vi "Colum_Auto_Size.vi"(8 "error in (no error)":errorcluster, 10 "Table With header":string[][](array[string])=[["", ""], ["", ""]], 11 "Table reference":refnum<vi>) -> (0 "error out":errorcluster)   [LabVIEW 2017]
doc: "This Vi is Created by Asim Lambay for auto sizing of Table Colum. Please use header also with it."
uses:
  <vilib>/Utility/miscctls.llb/LVRowAndColumnTypeDef.ctl
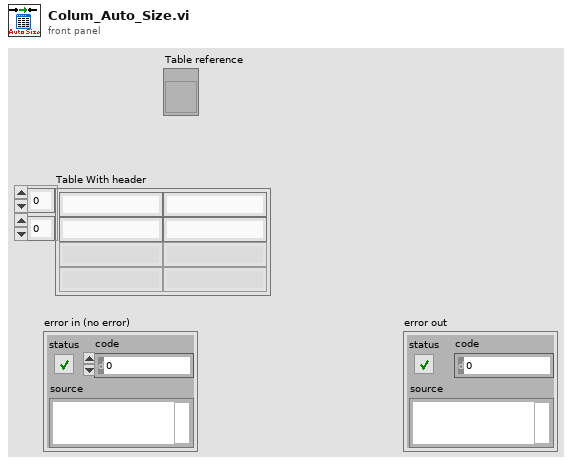
[diagram p1: front panel]
types:
  T1 = typedef "LVRowAndColumnTypeDef.ctl" = cluster{"Row":i32, "Column":i32}
  T2 = typedef "LVBoundsTypeDef.ctl" = cluster{"Width":u32, "Height":u32}
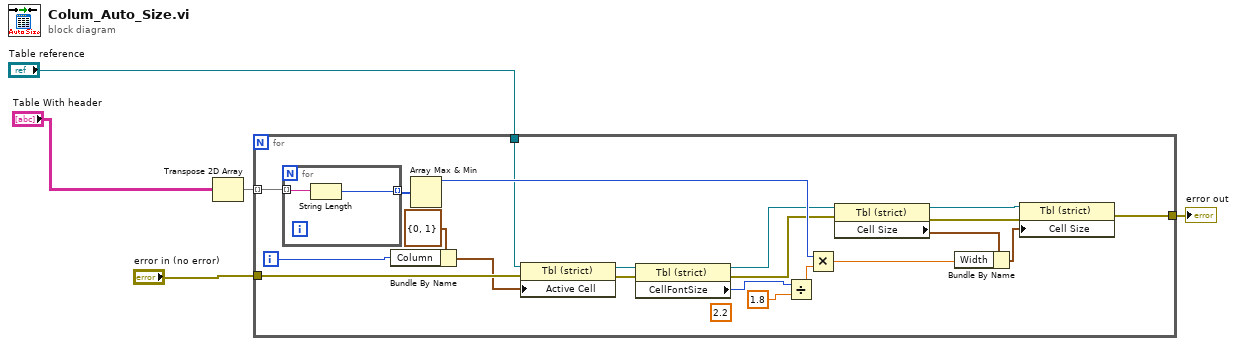
[diagram p0: block diagram]
diagram:
  n1 = Transpose 2D Array(2D array="Table With header") -> (transposed array=w4:string[][])
  n2 = for {
    tunnel: w4 -> [w26] mode=indexing
    tunnel: "error in (no error)" -> [w22]
    tunnel: [w8] -> w2
    tunnel: "Table reference" -> [w7]
    i -> [w23]
    (unwired) 2.2 ("x/y 2")
    n3 = for {
      tunnel: w26 -> [w28] mode=indexing
      tunnel: [w27] -> w25 mode=indexing
      n4 = String Length(string=w28) -> (length=w27:i32)
    }
    n5 = Bundle By Name(cluster=T1 {"Row"=0, "Column"=1} ("Active Cel"), "Column"=w23) -> (w21:T1)
    n6 = Array Max & Min(array=w25) -> (max value=w16:i32)  [unwired: 3 out]
    n7 = property on="Property Node" class="Tbl (strict)"(reference=w7, error in=w22, "Active Cell"=w21) -> (reference out=w20:refnum<vi>, error out=w19:errorcluster)
    n8 = property on="Property Node" class="Tbl (strict)"(reference=w20, error in=w19) -> (reference out=w12:refnum<vi>, error out=w11:errorcluster, "CellFontSize"=w18:u32)
    n9 = Divide(x=w18, y=1.8 ("x/y 2")) -> (x/y=w17:dbl)
    n10 = Multiply(x=w16, y=w17) -> (x*y=w10:dbl)
    n11 = property on="Property Node" class="Tbl (strict)"(reference=w12, error in=w11) -> (reference out=w13:refnum<vi>, error out=w14:errorcluster, "Cell Size"=w15:T2)
    n12 = Bundle By Name(cluster=w15, "Width"=w10) -> (w9:T2)
    n13 = property on="Property Node" class="Tbl (strict)"(reference=w13, error in=w14, "Cell Size"=w9) -> (error out=w8:errorcluster)  [unwired: 1 out]
  }
  "error out" <- w2
